vi "Delete from Array (Single).vi"(8 "index":i32, 11 "LVJSON.lvlib:JSON Array In":refnum<class "JSON Array.lvclass">) -> (1 "deleted portion":refnum<class "JSON Null.lvclass">, 3 "JSON Array w/ subset deleted":refnum<class "JSON Array.lvclass">)   [LabVIEW 2015, in "LVJSON.lvlib" / "JSON Array.lvclass"]
uses:
  JSON Array.lvclass
  JSON Datatype/JSON Null.lvclass
  JSON Array.lvclass/JSON Array.ctl
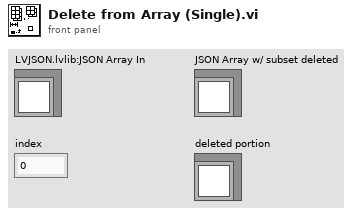
[diagram p1: front panel]
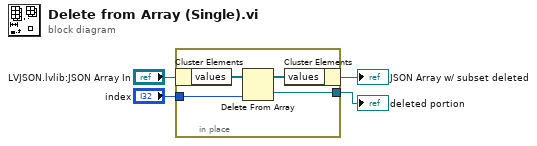
[diagram p0: block diagram]
diagram:
  n1 = in-place {
    in-place-border: "index" -> [w8]
    in-place-border: [w7] -> w1
    n2 = in-place-cluster #1("LVJSON.lvlib:JSON Array In") -> ("values"=w6:refnum<class "JSON Null.lvclass">[])
    n3 = Delete From Array(array=w6, index=w8) -> (deleted portion=w7:refnum<class "JSON Null.lvclass">, array with subset deleted=w5:refnum<class "JSON Null.lvclass">[])  [unwired: 1 in]
    n4 = in-place-cluster #1("values"=w5) -> (→"JSON Array w/ subset deleted":refnum<class "JSON Array.lvclass">)
  }
  "deleted portion" <- w1
